vi "Open MB.vi"(8 "error in (no error)":errorcluster, 11 "DAM0404D in":refnum<class "DAM0404D.lvclass">) -> (0 "error out":errorcluster, 3 "DAM0404D out":refnum<class "DAM0404D.lvclass">)   [LabVIEW 2016, in "DAM0404D.lvlib" / "DAM0404D.lvclass"]
uses:
  DAM0404D.lvclass
  <vilib>/Plasmionique/MB Master/MB_Master/MB_Master.lvclass
  DAM0404D.lvclass/DAM0404D.ctl
  <vilib>/Plasmionique/MB Master/MB_Master_Serial/MB_Master_Serial.lvclass
  C:/Program Files (x86)/National Instruments/LabVIEW 2016/vi.lib/Plasmionique/MB Master/MB_Master/MB_Master.lvclass
  <vilib>/Plasmionique/MB Master/MB_Master_TCP/MB_Master_TCP.lvclass
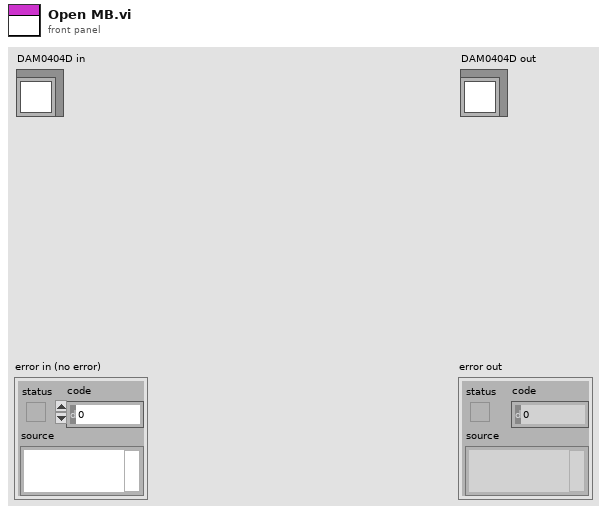
[diagram p1: front panel]
types:
  T1 = cluster{"baud rate (bps)":u32, "stop bits":u16, "parity":u16, "flow control":u16, "timeout":u32, "retries":i32}
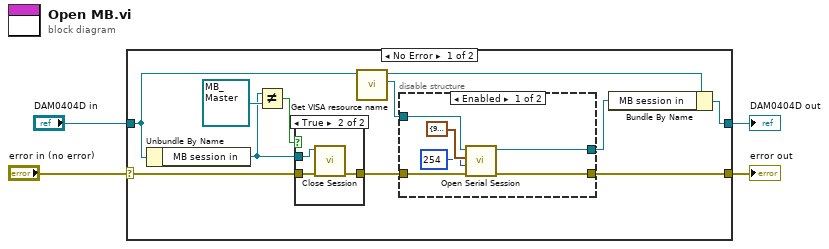
[diagram p0: block diagram]
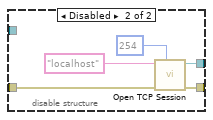
[diagram p2: hidden frame]
diagram:
  n1 = case shown="No Error" "error in (no error)" {
    selector: "error in (no error)" -> [w6 w32]
    tunnel: [w11 w32] -> w3
    tunnel: [w13 w31] -> w1
    tunnel: "DAM0404D in" -> [w10 w31]
    frame No Error {
      n2 = Unbundle By Name(w10) -> ("MB session in"=w8:refnum<class "MB_Master.lvclass">)
      n3 = Not Equal?(x=w8, y=refnum<class "MB_Master.lvclass"> refnum ("MB session in")) -> (x != y?=w7:bool)
      n4 = case shown="True" w7 {
        tunnel: w8 -> [_ w30]
        tunnel: w6 -> [w27 w29]
        tunnel: [w27 w28] -> w5
        frame False {
        }
        frame True {
          n5 = call-dynamic "Close Session.vi"("error in (no error)"=w29, "MB session in"=w30) -> ("error out"=w28:errorcluster)  [unwired: 9 in]
        }
      }
      n6 = call "Get VISA resource name.vi"("DAM0404D in"=w10) -> ("VISA resource name"=w14:refnum<visa-resource-name>, "DAM0404D out"=w15:refnum<class "DAM0404D.lvclass">)  [unwired: 9 in]
      n7 = disable-structure shown="Enabled" {
        disable-tunnel: w14 -> [w21 _]
        disable-tunnel: [w18 w26] -> w12
        disable-tunnel: [w17 w24] -> w11
        disable-tunnel: w5 -> [w16 w25]
        frame Enabled {
          n8 = call <vilib>:"Open Serial Session.vi"("Error in"=w16, "Slave ID"=u8 254, "Serial Config"=T1 {"baud rate (bps)"=9600, "stop bits"=10, "parity"=0, "flow control"=0, "timeout"=1000, "retries"=3}, "VISA Resource"=w21) -> ("Error out"=w17:errorcluster, "MB_Serial session"=w18:refnum<class "MB_Master_Serial.lvclass">)  [unwired: 6 in]
        }
        frame Disabled {
          n9 = call <vilib>:"Open TCP Session.vi"("Slave ID (255)"=u8 254, "error in (no error)"=w25, "IP Address"="localhost") -> ("error out"=w24:errorcluster, "MB_TCP session"=w26:refnum<class "MB_Master_TCP.lvclass">)  [unwired: 7 in]
        }
      }
      n10 = Bundle By Name(cluster=w15, "MB session in"=w12) -> (w13:refnum<class "DAM0404D.lvclass">)
    }
    frame Error {
    }
  }
  "error out" <- w3
  "DAM0404D out" <- w1
